vi "Setup.vi"(11 "Hello World Event in":refnum<class "Hello World Event.lvclass">) -> (3 "Hello World Event out":refnum<class "Hello World Event.lvclass">)   [LabVIEW 2021, in "Hello World Event.lvlib" / "Hello World Event.lvclass"]
uses:
  Hello World Event.lvclass
  Hello World Event.lvclass/Hello World Event.ctl
  <vilib>/Nathan Davis/jettl/jettl/Event/Event.lvclass
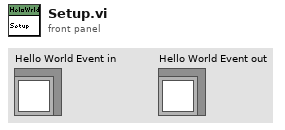
[diagram p1: front panel]
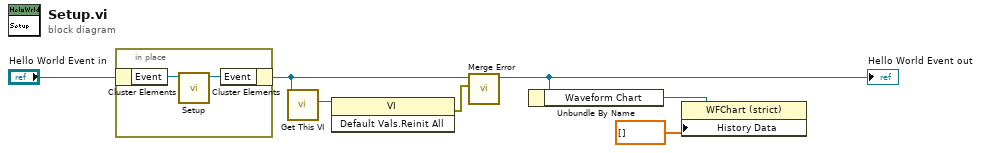
[diagram p0: block diagram]
diagram:
  n1 = in-place {
    n2 = in-place-cluster #1("Hello World Event in") -> ("Event"=w9:refnum<class "Event.lvclass">)
    n3 = call-dynamic "Setup.vi"("Setup in"=w9) -> ("Setup out"=w8:refnum<class "Event.lvclass">)  [unwired: 10 in]
    n4 = in-place-cluster #1("Event"=w8) -> (w4:refnum<class "Hello World Event.lvclass">)
  }
  n5 = call-dynamic "Get This VI.vi"("Hello World Event in"=w4) -> ("This VI"=w6:refnum<vi>)  [unwired: 10 in]
  n6 = invoke class="VI" method="Default Vals.Reinit All"(reference=w6) -> (error out=w5:errorcluster)  [unwired: 2 in, 2 out]
  n7 = call-dynamic "Merge Error.vi"("Error"=w5, "Hello World Event in"=w4) -> ("Hello World Event out"=w3:refnum<class "Hello World Event.lvclass">)  [unwired: 9 in]
  "Hello World Event out" <- w3
  n8 = Unbundle By Name(w3) -> ("Waveform Chart"=w2:refnum<vi>)
  n9 = property class="WFChart (strict)"(reference=w2, "History Data"=dbl[] []) -> ()  [unwired: 1 in, 2 out]
